vi "Calibrate Temperature 2 Ticks (uSMC).vi"(1 "SMindex":i32, 2 "temperature (Cels)":dbl) -> (0 "Temperature (ticks)":u16)   [LabVIEW 2010, in "SignalWriterMH110203USBStepperMotor.lvclass"]
uses:
  SignalWriterMH110203USBStepperMotor.lvclass
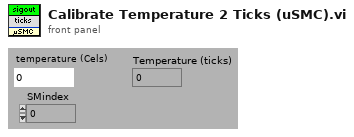
[diagram p1: front panel]
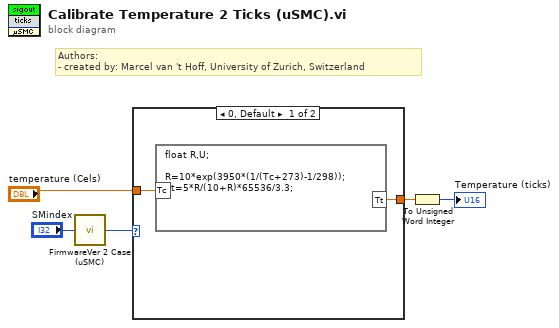
[diagram p0: block diagram]
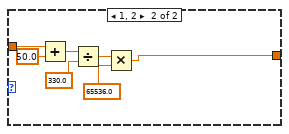
[diagram p2: hidden frame]
diagram:
  # "Authors: \n- created by: Marcel van 't Hoff, University of Zurich, Switzerland"
  n1 = call "FirmwareVer 2 Case (uSMC).vi"("SMindex"="SMindex") -> ("Case"=w2:i32)
  n2 = case shown="0, Default" w2 {
    tunnel: "temperature (Cels)" -> [w7 w14]
    tunnel: [w6 w8] -> w4
    frame 0, Default {
      n3 = formula code="float R,U;\n\nR=10*exp(3950*(1/(Tc+273)-1/298));\nTt=5*R/(10+R)*65536/3.3;"("Tc"=w7) -> ("Tt"=w6:dbl)
    }
    frame 1, 2 {
      n4 = Add(x=w14, y=50.0) -> (x+y=w12:dbl)
      n5 = Divide(x=w12, y=330.0) -> (x/y=w10:dbl)
      n6 = Multiply(x=w10, y=65536.0) -> (x*y=w8:dbl)
    }
  }
  n7 = To Unsigned Word Integer(number=w4) -> (unsigned 16bit integer=→"Temperature (ticks)":u16)
